vi "WLAN_SigContent.vi"(8 "error in (no error)":errorcluster, 10 "Frequency channel estimation":cdb[](array[numeric]) format="%.6g", 11 "SIG":cdb[](array[numeric])) -> (0 "error out":errorcluster, 1 "Symbol numbers":i32, 2 "encoded bit numbers":u32, 3 "original bit numbers":u32, 4 "Modulation parameter":T1, 5 "SIG valid?":bool)   [LabVIEW 2022 SP3]
panel:
  out "size(s) 2":i32
  out "size(s)":i32
  out "output bit stream":i8[](array[numeric])
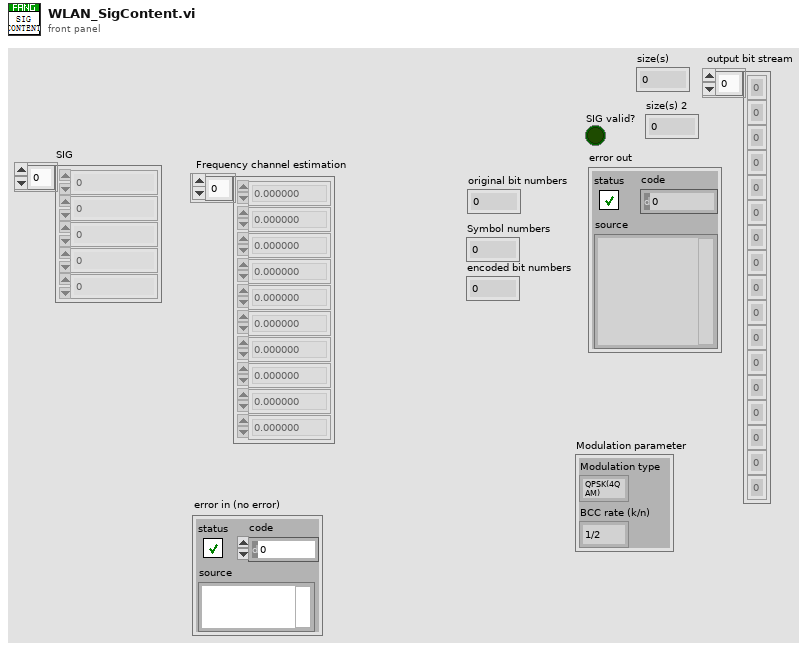
[diagram p1: front panel]
types:
  T1 = cluster{"Modulation type":enum16{"QPSK(4QAM)", "64QAM", "16QAM", "BPSK"}, "BCC rate (k/n)":enum16{"1/2", "2/3", "3/4"}}
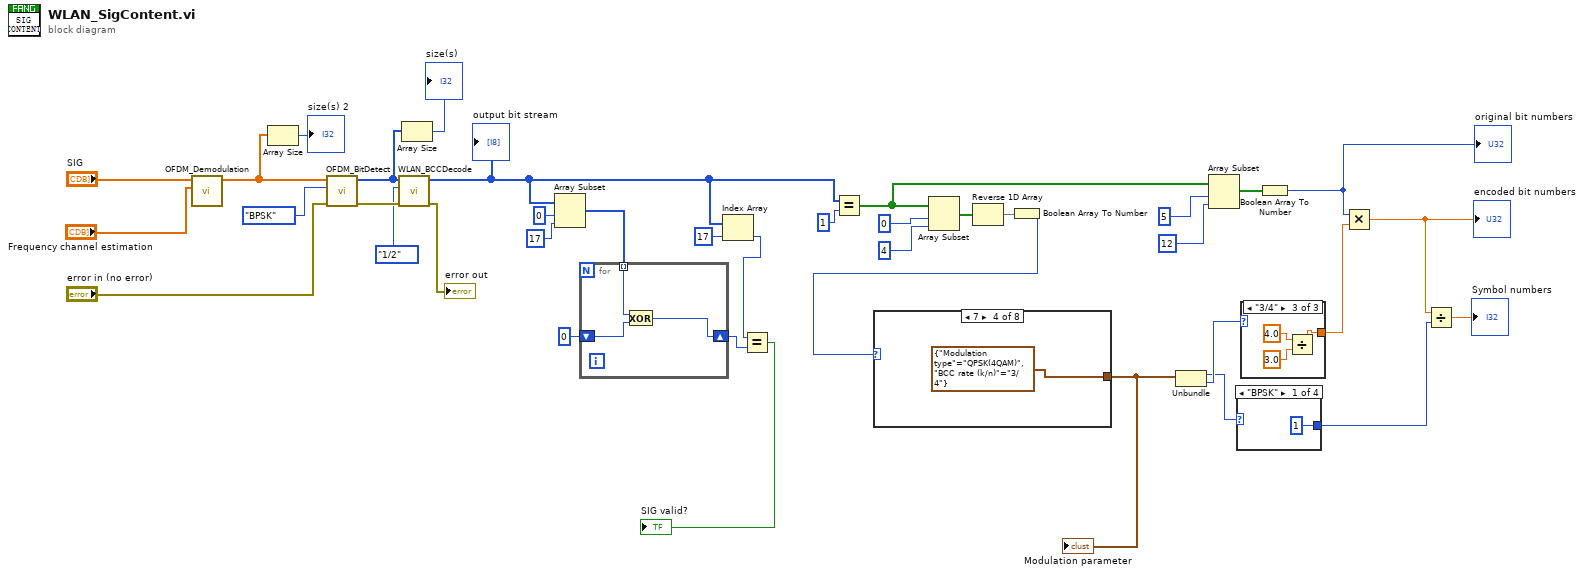
[diagram p0: block diagram]
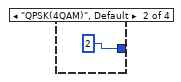
[diagram p2: hidden frame]
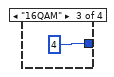
[diagram p3: hidden frame]
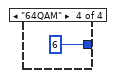
[diagram p4: hidden frame]
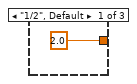
[diagram p5: hidden frame]
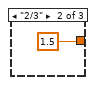
[diagram p6: hidden frame]
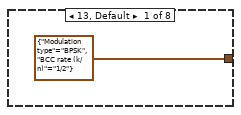
[diagram p7: hidden frame]
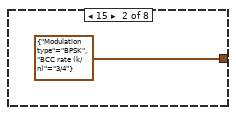
[diagram p8: hidden frame]
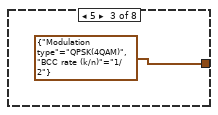
[diagram p9: hidden frame]
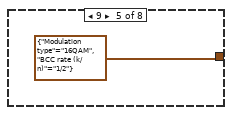
[diagram p10: hidden frame]
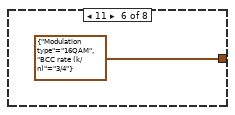
[diagram p11: hidden frame]
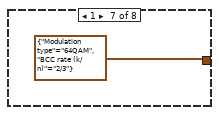
[diagram p12: hidden frame]
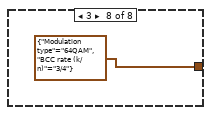
[diagram p13: hidden frame]
diagram:
  n1 = call "OFDM_Demodulation.vi"("Frequency channel estimation"="Frequency channel estimation", "Input sequence"="SIG") -> ("Output sequence"=w38:cdb[])  [unwired: 8 in, 1 out]
  n2 = Array Size(array=w38) -> (size(s)=→"size(s) 2":i32)
  n3 = call "OFDM_BitDetect.vi"("Input symbols"=w38, "Modulation type"=enum16{"QPSK(4QAM)", "64QAM", "16QAM", "BPSK"}."BPSK", "error in (no error)"="error in (no error)") -> ("Output bits"=w35:i8[], "error out"=w33:errorcluster)  [unwired: 6 in]
  n4 = call "WLAN_BCCDecode.vi"("error in (no error)"=w33, "BCC rate (k/n)"=enum16{"1/2", "2/3", "3/4"}."1/2", "input bit stream"=w35) -> ("error out"=→"error out":errorcluster, "output bit stream"=w29:i8[])  [unwired: 7 in]
  "output bit stream" <- w29
  n5 = Array Size(array=w35) -> (size(s)=→"size(s)":i32)
  n6 = Array Subset(array=w29, index=0, length=17) -> (w19:i8[])
  n7 = for {
    shift-right: [w40] -> w15
    shift-left: i8 0 -> [w41]
    tunnel: w19 -> [w39] mode=indexing
    n8 = Exclusive Or(1:w41, 2:w39) -> (0:w40:i8)
  }
  n9 = Index Array(array=w29, index=17) -> (element=w16:i8)
  n10 = Equal?(x=w16, y=w15) -> (x = y?=→"SIG valid?":bool)
  n11 = Equal?(x=w29, y=1 ("length")) -> (x = y?=w34:bool[])
  n12 = Array Subset(array=w34, index=0, length=4) -> (w10:bool[])
  n13 = Reverse 1D Array(array=w10) -> (reversed array=w9:bool[])
  n14 = Boolean Array To Number(Boolean array=w9) -> (number=w8:u32)
  n15 = case shown="7" w8 {
    tunnel: [T1 {"Modulation type"=enum."BPSK", "BCC rate (k/n)"=enum."1/2"} ("Modulation parameter") T1 {"Modulation type"=enum."BPSK", "BCC rate (k/n)"=enum."3/4"} ("Modulation parameter") T1 {"Modulation type"=enum."QPSK(4QAM)", "BCC rate (k/n)"=enum."1/2"} ("Modulation parameter") T1 {"Modulation type"=enum."QPSK(4QAM)", "BCC rate (k/n)"=enum."3/4"} ("Modulation parameter") T1 {"Modulation type"=enum."16QAM", "BCC rate (k/n)"=enum."1/2"} ("Modulation parameter") T1 {"Modulation type"=enum."16QAM", "BCC rate (k/n)"=enum."3/4"} ("Modulation parameter") T1 {"Modulation type"=enum."64QAM", "BCC rate (k/n)"=enum."2/3"} ("Modulation parameter") T1 {"Modulation type"=enum."64QAM", "BCC rate (k/n)"=enum."3/4"} ("Modulation parameter")] -> w28
    frame 13, Default {
    }
    frame 15 {
    }
    frame 5 {
    }
    frame 7 {
    }
    frame 9 {
    }
    frame 11 {
    }
    frame 1 {
    }
    frame 3 {
    }
  }
  "Modulation parameter" <- w28
  n16 = Unbundle(w28) -> ("Modulation type"=w3:enum16{"QPSK(4QAM)", "64QAM", "16QAM", "BPSK"}, "BCC rate (k/n)"=w4:enum16{"1/2", "2/3", "3/4"})
  n17 = Array Subset(array=w34, index=5, length=12) -> (w5:bool[])
  n18 = case shown="\"BPSK\"" w3 {
    tunnel: [1 2 4 6] -> w1
    frame "BPSK" {
    }
    frame "QPSK(4QAM)", Default {
    }
    frame "16QAM" {
    }
    frame "64QAM" {
    }
  }
  n19 = case shown="\"3/4\"" w4 {
    tunnel: [2.0 1.5 w58] -> w2
    frame "1/2", Default {
    }
    frame "2/3" {
    }
    frame "3/4" {
      n20 = Divide(x=4.0, y=3.0) -> (x/y=w58:dbl)
    }
  }
  n21 = Boolean Array To Number(Boolean array=w5) -> (number=w31:u32)
  "original bit numbers" <- w31
  n22 = Multiply(x=w31, y=w2) -> (x*y=w27:dbl)
  "encoded bit numbers" <- w27
  n23 = Divide(x=w27, y=w1) -> (x/y=→"Symbol numbers":dbl)
